vi "TestRFGVSummary.vi"() -> (0 "error out":errorcluster, 2 "Pass":bool)   [LabVIEW 2015]
uses:
  TypeDef/RequestActionEnum.ctl
  LVClasses/Request/PersonnelType.ctl
  LVClasses/Request/Request.lvclass
panel:
  out "Index":i32
  out "DataInit PUIDs":string
  out "Add Request 2":string
  out "Summary 2":string
  out "Add Request":string
  out "Read Requests":string
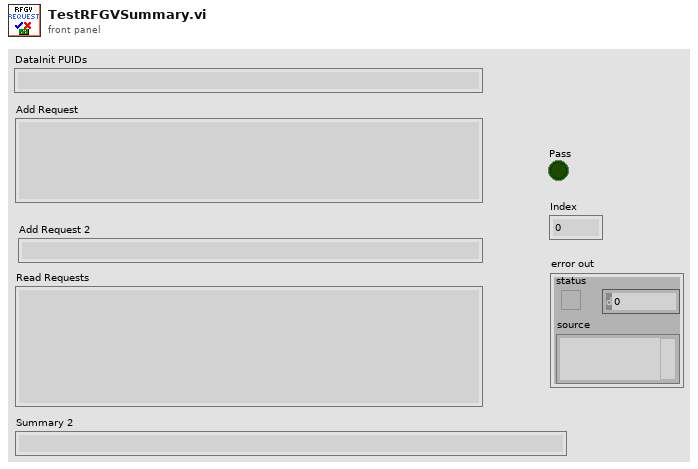
[diagram p1: front panel]
types:
  T1 = typedef "RequestActionEnum.ctl" = enum16{"Init", "ReadRequests", "ReadRequest", "AddRequest", "RemoveRequest", "ToDisk", "Ack", "Complete", "Read Summary"}
  T2 = typedef "Request.lvclass/PersonnelType.ctl" = u16
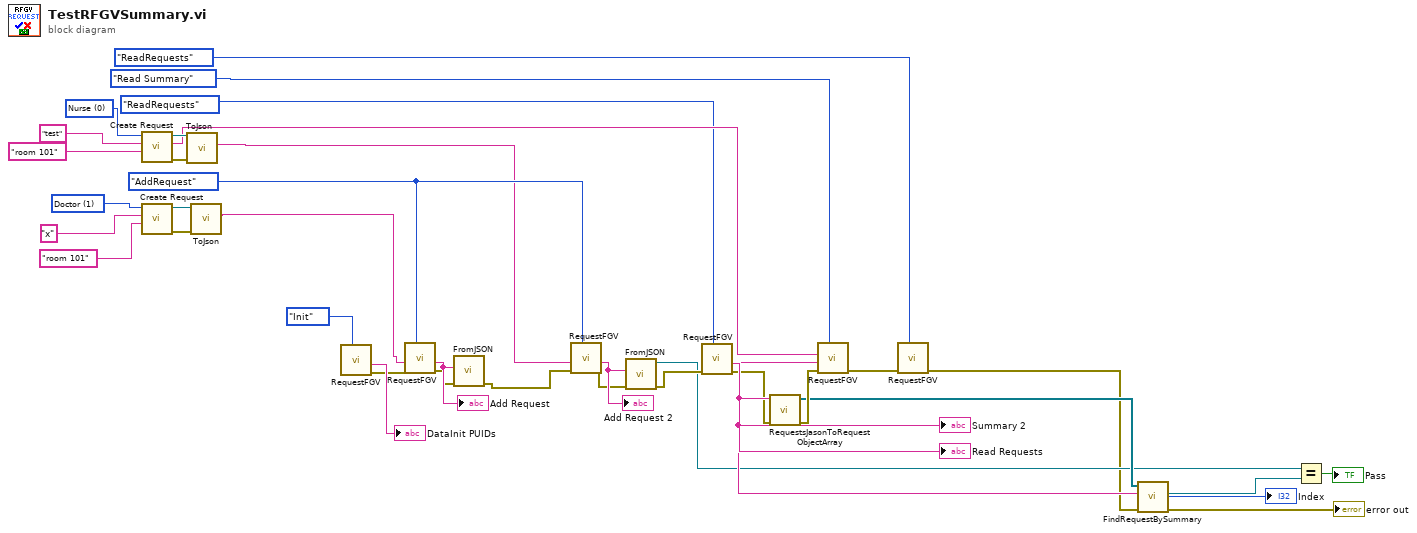
[diagram p0: block diagram]
diagram:
  w23 = T2 1 items=["Nurse", "Doctor", "Cleanning", "Admin"] ("Type 2")
  w26 = T2 0 items=["Nurse", "Doctor", "Cleanning", "Admin"] ("Type")
  w36 = RequestActionEnum."AddRequest" ("Actions")
  n1 = call "Create Request.vi"("Description"="room 101" (".Description"), "Name"="test", "Personnel Type"=w26) -> ("error out"=w31:errorcluster, "RUID"=w29:string, "Request out"=w35:refnum<class "Request.lvclass">)  [unwired: 6 in]
  n2 = call "Create Request.vi"("Description"="room 101" (".Description 2"), "Name"="x" ("Name 2"), "Personnel Type"=w23) -> ("error out"=w33:errorcluster, "Request out"=w32:refnum<class "Request.lvclass">)  [unwired: 6 in, 1 out]
  n3 = call "ToJson.vi"("error in (no error)"=w31, "Request"=w35) -> ("Request"=w34:string)  [unwired: 8 in, 1 out]
  n4 = call "ToJson.vi"("error in (no error)"=w33, "Request"=w32) -> ("Request"=w30:string)  [unwired: 8 in, 1 out]
  n5 = call "RequestFGV.vi"("Actions"=RequestActionEnum."Init") -> ("error out"=w19:errorcluster, "Data Out"=→"DataInit PUIDs":string)  [unwired: 9 in]
  n6 = call "RequestFGV.vi"("Actions"=w36, "error in (no error)"=w19, "Data In"=w30) -> ("error out"=w13:errorcluster, "Data Out"=w18:string)  [unwired: 7 in]
  "Add Request" <- w18
  n7 = call "FromJSON.vi"("error in (no error)"=w13, "Request"=w18) -> ("error out"=w14:errorcluster)  [unwired: 8 in, 1 out]
  n8 = call "RequestFGV.vi"("Actions"=w36, "error in (no error)"=w14, "Data In"=w34) -> ("error out"=w15:errorcluster, "Data Out"=w17:string)  [unwired: 7 in]
  "Add Request 2" <- w17
  n9 = call "FromJSON.vi"("error in (no error)"=w15, "Request"=w17) -> ("error out"=w16:errorcluster, "Request out"=w5:refnum<class "Request.lvclass">)  [unwired: 8 in]
  n10 = call "RequestFGV.vi"("Actions"=RequestActionEnum."ReadRequests", "error in (no error)"=w16) -> ("error out"=w10:errorcluster, "Data Out"=w11:string)  [unwired: 8 in]
  "Read Requests" <- w11
  n11 = call "RequestsJasonToRequestObjectArray.vi"("error in (no error)"=w10, "Requests"=w11) -> ("error out"=w9:errorcluster, "REquests"=w8:refnum<class "Request.lvclass">[])  [unwired: 8 in]
  n12 = call "RequestFGV.vi"("Actions"=RequestActionEnum."Read Summary", "error in (no error)"=w9, "RUID"=w29) -> ("error out"=w12:errorcluster, "Data Out"=w7:string)  [unwired: 7 in]
  "Summary 2" <- w7
  n13 = call "RequestFGV.vi"("Actions"=RequestActionEnum."ReadRequests", "error in (no error)"=w12) -> ("error out"=w2:errorcluster)  [unwired: 8 in, 1 out]
  n14 = call "FindRequestBySummary.vi"("error in (no error)"=w2, "Request Summary"=w7, "Requests"=w8) -> ("error out"=→"error out":errorcluster, "Index"=→"Index":i32, "Request out"=w6:refnum<class "Request.lvclass">)  [unwired: 5 in, 1 out]
  n15 = Equal?(x=w5, y=w6) -> (x = y?=→"Pass":bool)
